vi "RotateArrayAndScaleX.vi"(1 "Scale":dbl=-1.0 format="%#_13g", 2 "Angle":dbl, 3 "X, Y, Z Input":dbl[](array[numeric])) -> (0 "c * X', Y', Z Output":dbl[](array[numeric]))   [LabVIEW 2016]
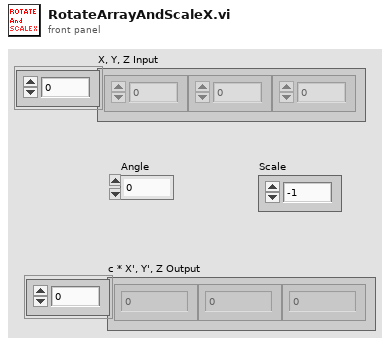
[diagram p1: front panel]
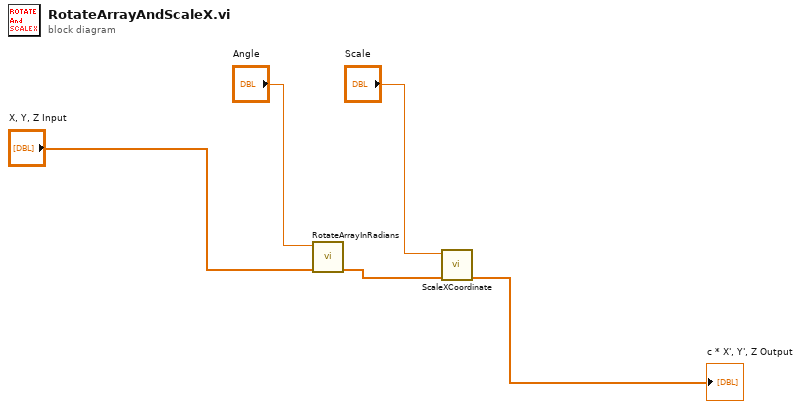
[diagram p0: block diagram]
diagram:
  n1 = call "RotateArrayInRadians.vi"("X, Y, Z Input"="X, Y, Z Input", "Angle"="Angle") -> ("X', Y', Z Output"=w2:dbl[])  [unwired: 9 in]
  n2 = call "ScaleXCoordinate.vi"("X, Y, Z Input"=w2, "Scale"="Scale") -> ("c * X, Y, Z Output"=→"c * X', Y', Z Output":dbl[])  [unwired: 9 in]
